vi "Update Test-Assertion Measurement.vi"(8 "error in (no error)":errorcluster, 9 "Measurement":refnum<class "TestManagerMsg.Measurement.lvclass">, 11 "Test Event Storage in":refnum<class "Test Event Storage.lvclass">) -> (0 "error out":errorcluster, 3 "Test Event Storage out":refnum<class "Test Event Storage.lvclass">)   [LabVIEW 2013, in "Caraya.lvlib" / "Test Event Storage.lvclass"]
uses:
  Test Event Storage.lvclass
  Test Manager Message Measurement/TestManagerMsg.Measurement.lvclass
  Test Event Storage.lvclass/Test Event Storage.ctl
  Test Result/Assert Event Data.ctl
  Test Manager Message/TestManagerMsg.lvclass/TestManagerMsg.ctl
  Test Manager Message Measurement/TestManagerMsg.Measurement.lvclass/TestManagerMsg.Measurement.ctl
  assert store -- cluster.ctl
  Test Manager Message Assertion/TestManagerMsg.Assertion.lvclass
  Test Manager Message Verbose/TestManagerMsg.Verbose.lvclass
  Test Manager Message/TestManagerMsg.lvclass
  Test Result/Test Result.lvclass
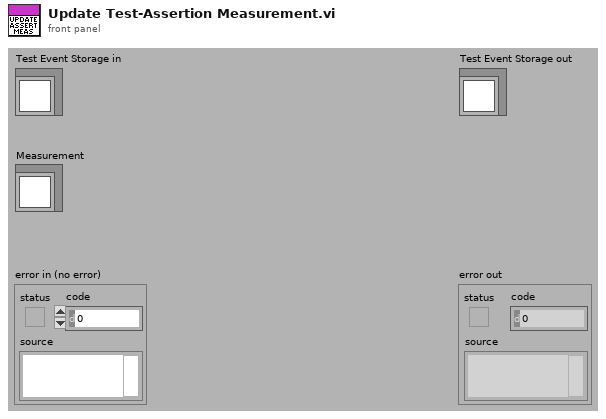
[diagram p1: front panel]
types:
  T1 = typedef "Caraya.lvlib/Test Result.lvclass/Assert Event Data.ctl" = cluster{"Name":string, "Passed":bool, "Call Chain":string[], "Test Error":errorcluster, "Time Stamp":timestamp, "Unique Assert ID":string, "Test ID":string, "Execution time (s)":dbl, "Verbose Explanation":string, "properties":variant, "measurements":variant, "limits":variant}
  T2 = typedef "Caraya.lvlib/Test Event Storage.lvclass/assert store -- cluster.ctl" = cluster{"Assertion":refnum<class "TestManagerMsg.Assertion.lvclass">, "Explanation":refnum<class "TestManagerMsg.Verbose.lvclass">, "properties":variant, "measurements":variant, "limits":variant}
  T3 = typedef "Caraya.lvlib/Test Event Storage.lvclass/store version -- enum.ctl" = enum16{"v1", "v2"}
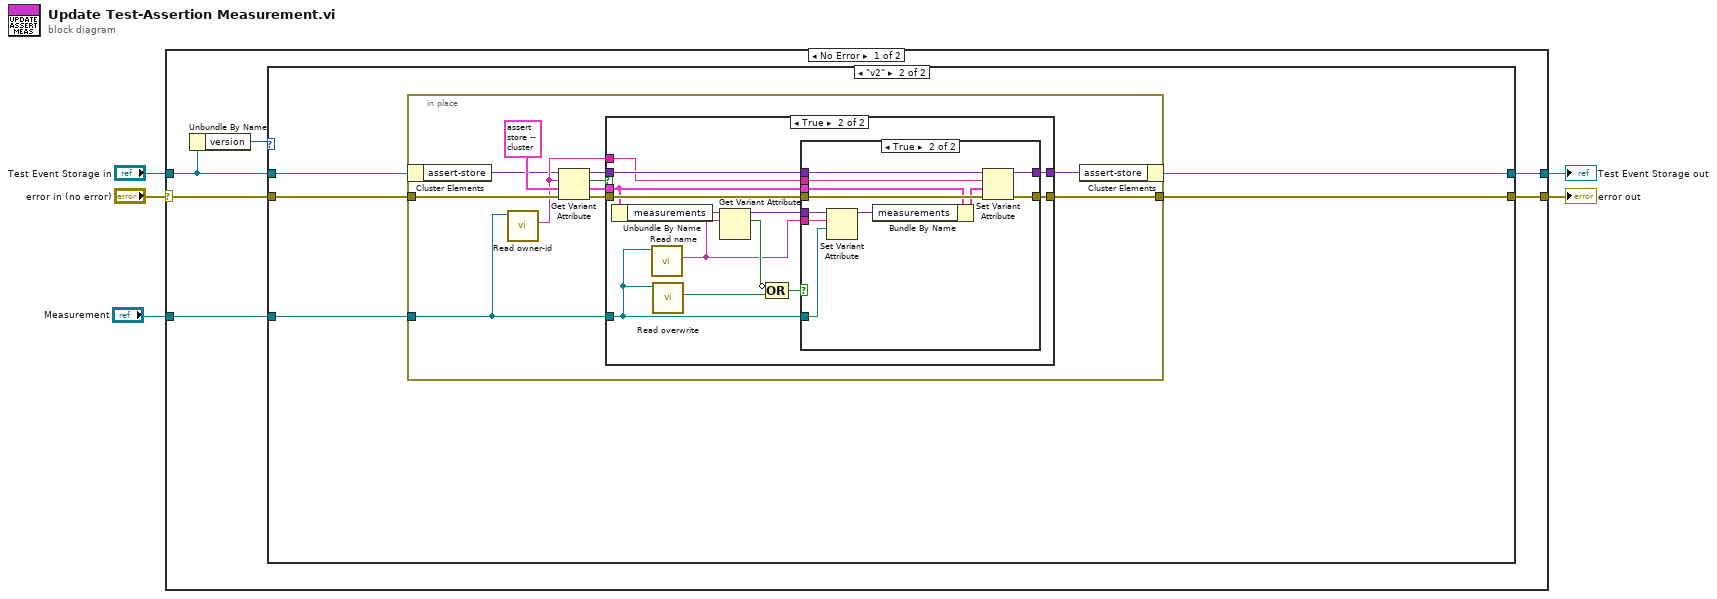
[diagram p0: block diagram]
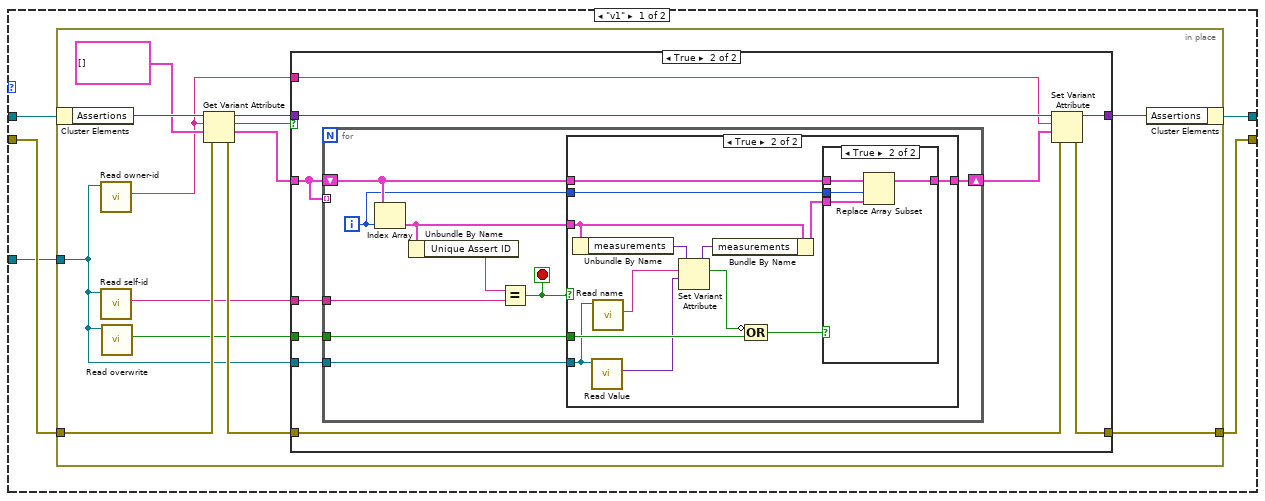
[diagram p2: hidden frame]
diagram:
  n1 = case shown="No Error" "error in (no error)" {
    selector: "error in (no error)" -> [w9 w115]
    tunnel: [w11 w115] -> w4
    tunnel: [w10 w114] -> w2
    tunnel: "Test Event Storage in" -> [w7 w114]
    tunnel: "Measurement" -> [w8 _]
    frame No Error {
      n2 = Unbundle By Name(w7) -> ("version"=w6:T3)
      n3 = case shown="\"v2\"" w6 {
        tunnel: [w16 w70] -> w11
        tunnel: [w15 w71] -> w10
        tunnel: w9 -> [w14 w73]
        tunnel: w8 -> [w13 w72]
        tunnel: w7 -> [w12 w74]
        frame "v1" {
          n4 = in-place {
            in-place-border: w14 -> [w23]
            in-place-border: [w28] -> w16
            in-place-border: w13 -> [w17]
            n5 = in-place-cluster #1(w12) -> ("Assertions"=w26:variant)
            n6 = call "Read owner-id.vi"("TestManagerMsg in"=w17) -> ("owner-id"=w19:string)  [unwired: 9 in, 1 out]
            n7 = call "Read self-id.vi"("TestManagerMsg in"=w17) -> ("self-id"=w20:string)  [unwired: 9 in, 1 out]
            n8 = call "Read overwrite.vi"("TestManagerMsg in"=w17) -> ("overwrite?"=w18:bool)  [unwired: 9 in, 1 out]
            n9 = Get Variant Attribute(Variant=w26, name=w19, default value (empty Variant)=T1[] [] ("Assertions"), error in=w23) -> (duplicate Variant=w27:variant, found=w25:bool, value=w24:T1[], error out=w22:errorcluster)
            n10 = case shown="True" w25 {
              tunnel: [w31 w41] -> w29
              tunnel: [w30 w40] -> w28
              tunnel: w22 -> [w30 w39]
              tunnel: w27 -> [w31 w38]
              tunnel: w19 -> [_ w37]
              tunnel: w24 -> [_ w32]
              tunnel: w17 -> [_ w36]
              tunnel: w20 -> [_ w34]
              tunnel: w18 -> [_ w33]
              frame False {
              }
              frame True {
                n11 = for {
                  tunnel: w36 -> [w50]
                  tunnel: w34 -> [w48]
                  tunnel: w33 -> [w47]
                  shift-right: [w49] -> w35
                  shift-left: w32 -> [w44]
                  tunnel: w32 -> [_] mode=indexing
                  i -> [w43]
                  stop <- w46 stop-if-true
                  n12 = Index Array(array=w44, index=w43) -> (element=w42:T1)
                  n13 = Unbundle By Name(w42) -> ("Unique Assert ID"=w45:string)
                  n14 = Equal?(x=w45, y=w48) -> (x = y?=w46:bool)
                  n15 = case shown="True" w46 {
                    tunnel: w50 -> [_ w53]
                    tunnel: [w51 w63] -> w49
                    tunnel: w44 -> [w51 w64]
                    tunnel: w47 -> [_ w57]
                    tunnel: w43 -> [_ w62]
                    tunnel: w42 -> [_ w61]
                    frame False {
                    }
                    frame True {
                      n16 = Unbundle By Name(w61) -> ("measurements"=w59:variant)
                      n17 = call "Read Value.vi"("TestManagerMsg.Measurement in"=w53) -> ("Value"=w52:variant)  [unwired: 9 in, 1 out]
                      n18 = call "Read name.vi"("TestManagerMsg.Measurement in"=w53) -> ("name"=w54:string)  [unwired: 9 in, 1 out]
                      n19 = Set Variant Attribute(Variant=w59, name=w54, value=w52) -> (Variant out=w58:variant, replaced=w56:bool)  [unwired: 1 in, 1 out]
                      n20 = Bundle By Name(cluster=w61, "measurements"=w58) -> (w60:T1)
                      n21 = Compound Arithmetic op=OR(invert w56, w57) -> (w55:bool)
                      n22 = case shown="True" w55 {
                        tunnel: w64 -> [w65 w69]
                        tunnel: [w65 w68] -> w63
                        tunnel: w62 -> [_ w67]
                        tunnel: w60 -> [_ w66]
                        frame False {
                        }
                        frame True {
                          n23 = Replace Array Subset(array=w69, new element=w66, index=w67) -> (w68:T1[])
                        }
                      }
                    }
                  }
                }
                n24 = Set Variant Attribute(Variant=w38, name=w37, value=w35, error in=w39) -> (Variant out=w41:variant, error out=w40:errorcluster)  [unwired: 1 out]
              }
            }
            n25 = in-place-cluster #1("Assertions"=w29) -> (w15:refnum<class "Test Event Storage.lvclass">)
          }
        }
        frame "v2" {
          n26 = in-place {
            in-place-border: w73 -> [w83]
            in-place-border: [w84] -> w70
            in-place-border: w72 -> [w82]
            n27 = in-place-cluster #2(w74) -> ("assert-store"=w75:variant)
            n28 = call "Read owner-id.vi"("TestManagerMsg in"=w82) -> ("owner-id"=w76:string)  [unwired: 9 in, 1 out]
            n29 = Get Variant Attribute(Variant=w75, name=w76, default value (empty Variant)=T2 {"Assertion"=refnum, "Explanation"=refnum, "properties"=variant, "measurements"=variant, "limits"=variant} ("assert-store"), error in=w83) -> (duplicate Variant=w81:variant, found=w80:bool, value=w79:T2, error out=w78:errorcluster)
            n30 = case shown="True" w80 {
              tunnel: [w87 w100] -> w85
              tunnel: [w86 w99] -> w84
              tunnel: w78 -> [w86 w98]
              tunnel: w81 -> [w87 w97]
              tunnel: w76 -> [_ w96]
              tunnel: w79 -> [_ w95]
              tunnel: w82 -> [_ w89]
              frame False {
              }
              frame True {
                n31 = Unbundle By Name(w95) -> ("measurements"=w93:variant)
                n32 = call "Read name.vi"("TestManagerMsg.Measurement in"=w89) -> ("name"=w88:string)  [unwired: 9 in, 1 out]
                n33 = call "Read overwrite.vi"("TestManagerMsg in"=w89) -> ("overwrite?"=w91:bool)  [unwired: 9 in, 1 out]
                n34 = Get Variant Attribute(Variant=w93, name=w88) -> (duplicate Variant=w90:variant, found=w92:bool)  [unwired: 2 in, 2 out]
                n35 = Compound Arithmetic op=OR(invert w92, w91) -> (w94:bool)
                n36 = case shown="True" w94 {
                  tunnel: [w102 w113] -> w100
                  tunnel: [w101 w112] -> w99
                  tunnel: w98 -> [w101 w111]
                  tunnel: w97 -> [w102 w110]
                  tunnel: w96 -> [_ w109]
                  tunnel: w95 -> [_ w108]
                  tunnel: w89 -> [_ w103]
                  tunnel: w90 -> [_ w105]
                  tunnel: w88 -> [_ w104]
                  frame False {
                  }
                  frame True {
                    n37 = Set Variant Attribute(Variant=w105, name=w104, value=w103) -> (Variant out=w106:variant)  [unwired: 1 in, 2 out]
                    n38 = Bundle By Name(cluster=w108, "measurements"=w106) -> (w107:T2)
                    n39 = Set Variant Attribute(Variant=w110, name=w109, value=w107, error in=w111) -> (Variant out=w113:variant, error out=w112:errorcluster)  [unwired: 1 out]
                  }
                }
              }
            }
            n40 = in-place-cluster #2("assert-store"=w85) -> (w71:refnum<class "Test Event Storage.lvclass">)
          }
        }
      }
    }
    frame Error {
    }
  }
  "error out" <- w4
  "Test Event Storage out" <- w2
